vi "Create Download Initiate Response Message.vi"(11 "Service Data Object in":refnum<class "Service Data Object.lvclass">) -> (2 "CANopen Response Message":refnum<class "CANopen Response Message.lvclass">, 3 "Service Data Object out":refnum<class "Service Data Object.lvclass">)   [LabVIEW 2024, in "CANopen Master.lvlib" / "Service Data Object.lvclass"]
uses:
  Service Data Object.lvclass
  Service Data Object.lvclass/Service Data Object.ctl
  CANopen/FunctionCode.ctl
  CANopen Master.lvlib
  CANopen Message/CANopen Message.lvclass
  CANopen Response/CANopen Response Message.lvclass
  D:/git/CANopen-XNET/CANopen Message/CANopen Message.lvclass
  D:/git/CANopen-XNET/CANopen Response/CANopen Response Message.lvclass
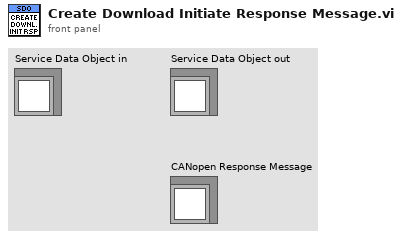
[diagram p1: front panel]
types:
  T1 = typedef "CANopen Master.lvlib/FunctionCode.ctl" = u16
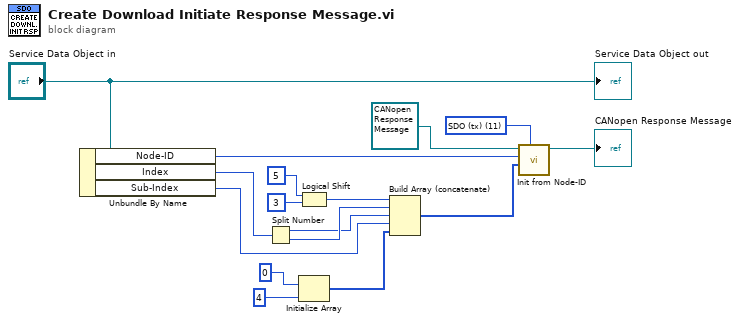
[diagram p0: block diagram]
diagram:
  w4 = T1 11 items=["EMCY"=1, "PDO1 (tx)"=3, "PDO1 (rx)"=4, "PDO2 (tx)"=5, "PDO2 (rx)"=6, "PDO3 (tx)"=7, "PDO3 (rx)"=8, "PDO4 (tx)"=9, "PDO4 (rx)"=10, "SDO (tx)"=11, "SDO (rx)"=12, "NMT error control"=14] ("Function code")
  n1 = Unbundle By Name("Service Data Object in") -> ("Node-ID"=w5:u8, "Index"=w12:u16, "Sub-Index"=w9:u8)
  n2 = Split Number(x=w12) -> (hi(x)=w10:u8, lo(x)=w11:u8)
  n3 = Logical Shift(y=5 ("x"), x=u8 3) -> (x << y=w14:u8)
  n4 = Initialize Array(u8 0, 4 ("dimension size")) -> (w7:u8[])
  n5 = Build Array (concatenate)(w14, w11, w10, w9, w7) -> (w3:u8[])
  n6 = call "Init from Node-ID.vi"("Function code"=w4, "Data"=w3, "Node-ID"=w5, "CANopen Message in"=refnum<class "CANopen Response Message.lvclass"> refnum ("CANopen Master.lvlib:CANopen Response Message.lvclass")) -> ("CANopen Message in"=→"CANopen Response Message":refnum<class "CANopen Response Message.lvclass">)  [unwired: 7 in]
  "Service Data Object out" <- "Service Data Object in"
